vi "dvp Vi Get Color Solution Sel Detail.vi"(7 "pIndex":i32, 9 "pColorSolutionSelstr":string, 10 "ColorSolutionSel":u32, 11 "handle":u32) -> (1 "pColorSolutionSelstr out":string, 3 "function return":u32(ring), 5 "pIndex out":i32)   [LabVIEW 2018, in "LabViewDVPCamera.lvlib"]
doc: "LabviewDvp2Api dvpStatus dvpViGetColorSolutionSelDetail(dvpHandle handle, dvpUint32 ColorSolutionSel, char *pColorSolutionSelstr, dvpInt32 *pIndex);"
uses:
  LabViewDVPCamera.lvlib
  LabViewDVPCamera/LabViewDVPCamera.dll
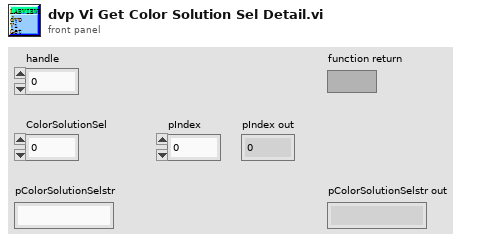
[diagram p1: front panel]
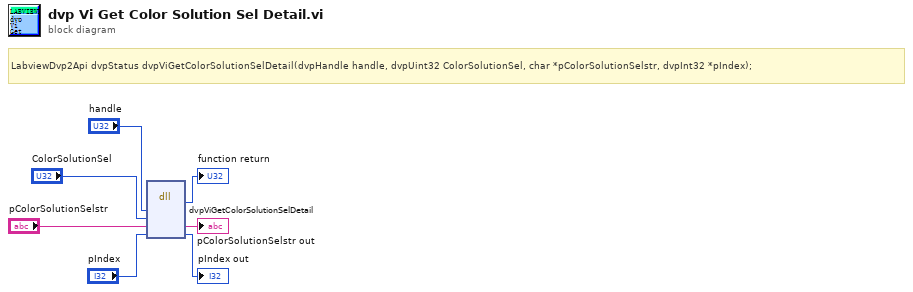
[diagram p0: block diagram]
diagram:
  # "LabviewDvp2Api dvpStatus dvpViGetColorSolutionSelDetail(dvpHandle handle, dvpUint32 ColorSolutionSel, char *pColorSolutionSelstr, dvpInt32 *pIndex);"
  n1 = dll-call lib="C:/Program Files (x86)/DVP2 Labview cn 64/Sample/LabViewDVPCamera/LabViewDVPCamera.*" fn="dvpViGetColorSolutionSelDetail"("handle"="handle", "ColorSolutionSel"="ColorSolutionSel", "pColorSolutionSelstr"="pColorSolutionSelstr", "pIndex"="pIndex") -> (→"function return":u32, "pColorSolutionSelstr"=→"pColorSolutionSelstr out":string, "pIndex"=→"pIndex out":i32)  [unwired: 5 in, 2 out]
